vi "Get Audio File Info.vi"(8 "error in (no error)":errorcluster, 10 "Codec":string, 11 "Path In":path) -> (0 "error out":errorcluster, 1 "Audio File Info":T1, 2 "Sample Length":u64, 3 "Path Out":path)   [LabVIEW 2020, in "G-Audio.lvlib"]
doc: "Retrieve audio file information. Some codecs (mp3) require the entire file be parsed to accuractely determine the length, which can take time for very large files. If <b>codec</b> isn't specified, file extension determines the codec type.\n\nSupported codecs: flac, mp3, ogg (vorbis), and wav."
uses:
  G-Audio.lvlib
  Controls/Audio File Info.ctl
  Private/Get File Extension (Reentrant).vi
  <vilib>/Utility/error.llb/Error Cluster From Error Code.vi
  lib/g_audio_x86.dll
  lib/g_audio_x64.dll
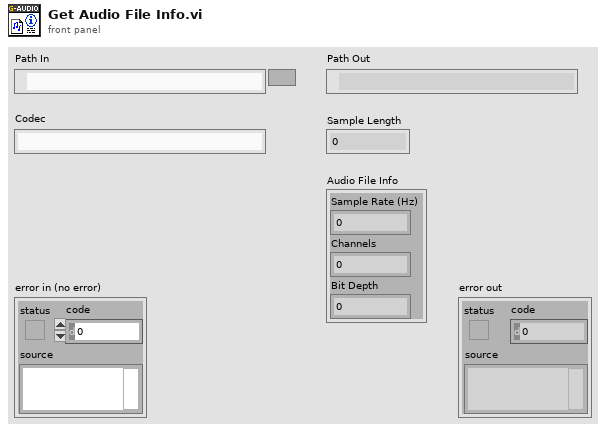
[diagram p1: front panel]
types:
  T1 = typedef "G-Audio.lvlib/Audio File Info.ctl" = cluster{"Sample Rate (Hz)":u32, "Channels":u32, "Bit Depth":u32}
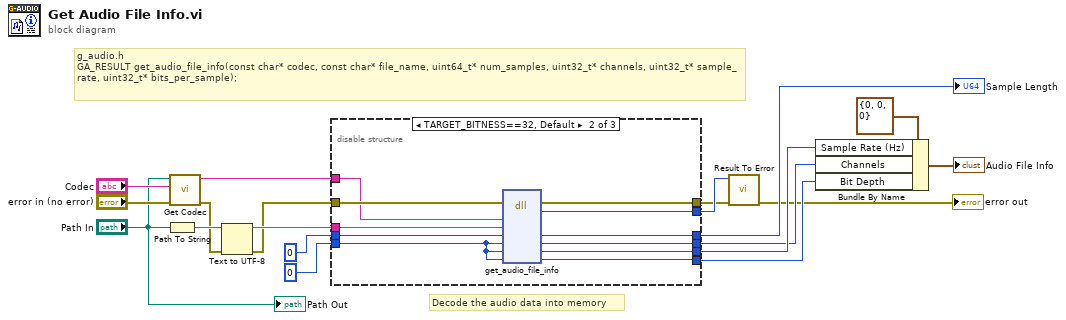
[diagram p0: block diagram]
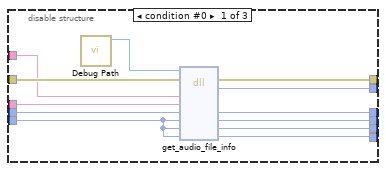
[diagram p2: hidden frame]
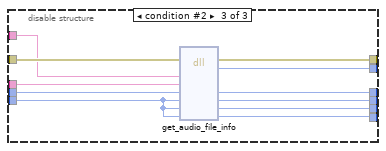
[diagram p3: hidden frame]
diagram:
  # "g_audio.h\nGA_RESULT get_audio_file_info(const char* codec, const char* file_name, uint64_t* num_samples, uint32_t* channels, uint32_t* sample_rate, uint32_t* bits_per_sample);"
  # "Decode the audio data into memory"
  n1 = Path To String(path="Path In") -> (string=w5:string)
  n2 = call "Get Codec.vi"("error in (no error)"="error in (no error)", "Codec In"="Codec", "Absolute Path"="Path In") -> ("error out"=w3:errorcluster, "Codec Out"=w9:string)  [unwired: 7 in]
  n3 = Text to UTF-8(8:w3, 11:w5) -> (0:w2:errorcluster, 3:w4:string)  [unwired: 1 in]
  n4 = disable-structure shown="TARGET_BITNESS==32, Default" {
    disable-tunnel: w2 -> [w31 w42 w53]
    disable-tunnel: [w29 w40 w51] -> w17
    disable-tunnel: [w28 w39 w50] -> w13
    disable-tunnel: [w27 w38 w49] -> w14
    disable-tunnel: w4 -> [w26 w37 w48]
    disable-tunnel: [w30 w41 w52] -> w7
    disable-tunnel: u32 0 ("num_samples") -> [w23 w34 w45]
    disable-tunnel: u64 0 ("num_samples") -> [w25 w36 w47]
    disable-tunnel: w9 -> [w24 w35 w46]
    disable-tunnel: [w22 w33 w44] -> w15
    disable-tunnel: [w21 w32 w43] -> w8
    frame condition #0 {
      n5 = call "Debug Path.vi"() -> ("Debug Path"=w20:path)  [unwired: 11 in]
      n6 = dll-call lib="?" fn="get_audio_file_info"(path in=w20, error in=w31, "codec"=w24, "file_name"=w26, "num_samples"=w25, "channels"=w23, "sample_rate"=w23, "bits_per_sample"=w23) -> (error out=w30:errorcluster, "result"=w21:i32, "num_samples"=w29:u64, "channels"=w28:u32, "sample_rate"=w27:u32, "bits_per_sample"=w22:u32)  [unwired: 3 in, 1 out]
    }
    frame condition #1 (active) {
      n7 = dll-call lib="C:/github/dataflowg/g-audio/src/LabVIEW/G-Audio/lib/g_audio_x86.*" fn="get_audio_file_info"(error in=w42, "codec"=w35, "file_name"=w37, "num_samples"=w36, "channels"=w34, "sample_rate"=w34, "bits_per_sample"=w34) -> (error out=w41:errorcluster, "result"=w32:i32, "num_samples"=w40:u64, "channels"=w39:u32, "sample_rate"=w38:u32, "bits_per_sample"=w33:u32)  [unwired: 4 in, 1 out]
    }
    frame condition #2 {
      n8 = dll-call lib="C:/github/dataflowg/g-audio/src/LabVIEW/G-Audio/lib/g_audio_x64.*" fn="get_audio_file_info"(error in=w53, "codec"=w46, "file_name"=w48, "num_samples"=w47, "channels"=w45, "sample_rate"=w45, "bits_per_sample"=w45) -> (error out=w52:errorcluster, "result"=w43:i32, "num_samples"=w51:u64, "channels"=w50:u32, "sample_rate"=w49:u32, "bits_per_sample"=w44:u32)  [unwired: 4 in, 1 out]
    }
  }
  "Sample Length" <- w17
  n9 = call "Result To Error.vi"("error in (no error)"=w7, "Result Code"=w8) -> ("error out"=→"error out":errorcluster)  [unwired: 9 in]
  n10 = Bundle By Name(cluster=T1 {"Sample Rate (Hz)"=0, "Channels"=0, "Bit Depth"=0} ("Audio File Info"), "Sample Rate (Hz)"=w14, "Channels"=w13, "Bit Depth"=w15) -> (→"Audio File Info":T1)
  "Path Out" <- "Path In"
